vi "York DIHB - Measure Load Cell.vi"() -> ()   [LabVIEW 2020]
uses:
  <vilib>/ptbypt/NI_PtbyPt.lvlib
panel:
  out "Amplifier Voltage (V - 1 Second Avg.)":dbl format="%0.4f"
  in  "stop":bool
  out "Amplifier Output Voltage":dynamicdata(graph)
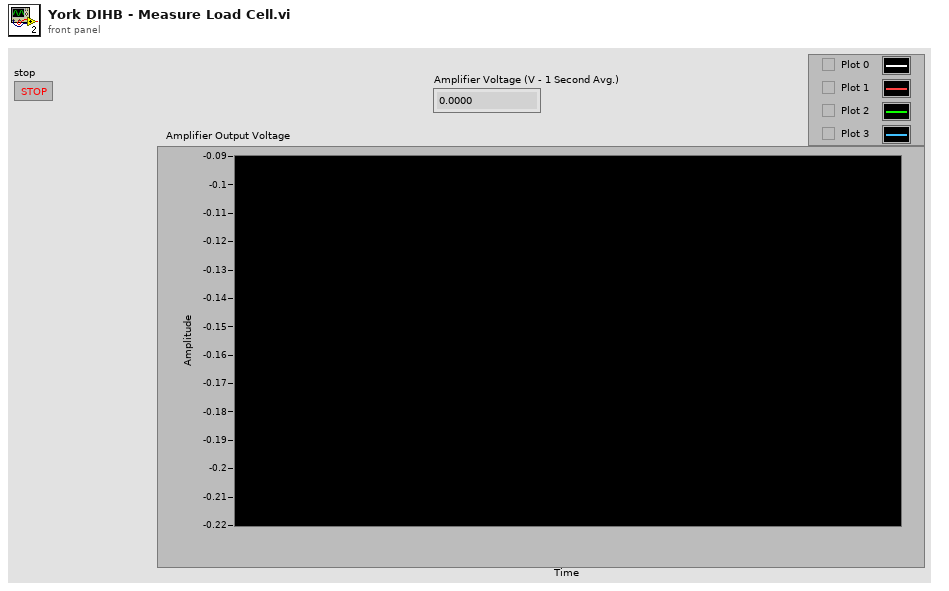
[diagram p1: front panel]
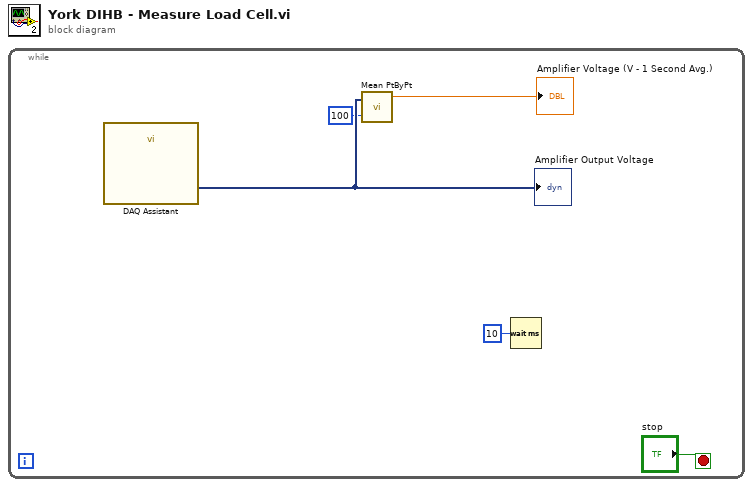
[diagram p0: block diagram]
diagram:
  n1 = while {
    stop <- "stop" stop-if-true
    n2 = call "DAQ Assistant"() -> ("data"=w3:dynamicdata)  [unwired: 17 in, 2 out]
    "Amplifier Output Voltage" <- w3
    n3 = call <vilib>:"Mean PtByPt.vi"("x"=w3, "sample length"=100) -> ("mean"=→"Amplifier Voltage (V - 1 Second Avg.)":dbl)  [unwired: 2 in, 1 out]
    n4 = Wait (ms)(milliseconds to wait=u32 10) -> ()  [unwired: 1 out]
  }
